vi "data_logging.vi"(11 "RowData":T1) -> ()   [LabVIEW 2019]
uses:
  RowData_Type.ctl
  store_last_RowData.vi
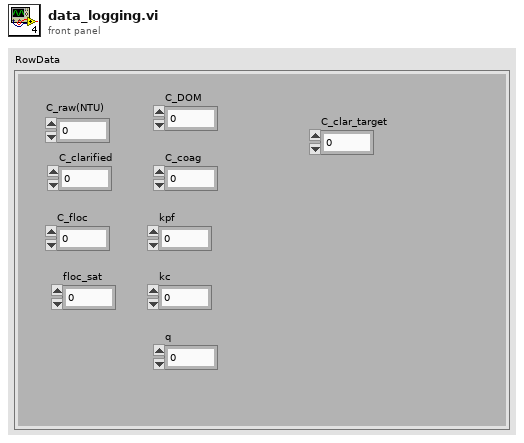
[diagram p1: front panel]
types:
  T1 = typedef "RowData_Type.ctl" = cluster{"C_raw(NTU)":dbl, "C_clarified":dbl, "C_floc":dbl, "floc_sat":dbl, "C_DOM":dbl, "C_coag":dbl, "kpf":dbl, "kc":dbl, "q":dbl, "C_clar_target":dbl}
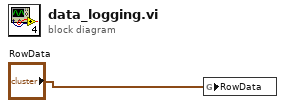
[diagram p0: block diagram]
diagram:
  n1 = global write "store_last_RowData.vi" "RowData"("RowData") -> ()
